vi "prepare_writing.vi"(8 "error in (no error)":errorcluster, 10 "fresh scan signals?":bool, 11 "DL090202ScanHead in":refnum<class "ScanHeadDL090202.lvclass">) -> (0 "error out":errorcluster, 3 "DL090202ScanHead out":refnum<class "ScanHeadDL090202.lvclass">)   [LabVIEW 2010, in "ScanHeadDL090202.lvclass"]
uses:
  ScanHeadDL090202.lvclass
  common/enumerations/functional_global_action_enum.ctl
  SignalWriter/GenericSignalWriter/GenericSignalWriter/GenericSignalWriter.lvclass
  Trajectory/TrajectoryDL091126GenericVoxel/TrajectoryDL091126GenericVoxel/TrajectoryDL091126GenericVoxel.lvclass
  ScanHeadDL090202.lvclass/ScanHeadDL090202.ctl
  Trajectory/GenericTrajectory/GenericTrajectory/GenericTrajectory.lvclass
  common/classes/GenericComponent/GenericComponent/class_data.vi
  common/classes/ErrorController/ErrorController/class_data.vi
  common/classes/ErrorController/ErrorController/ErrorController.lvclass
  common/classes/GenericComponent/GenericComponent/GenericComponent.lvclass
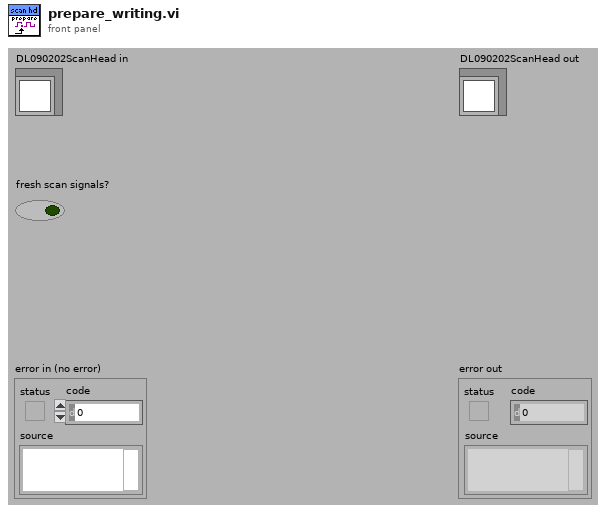
[diagram p1: front panel]
types:
  T1 = typedef "functional_global_action_enum.ctl" = enum16{"get", "set", "reset"}
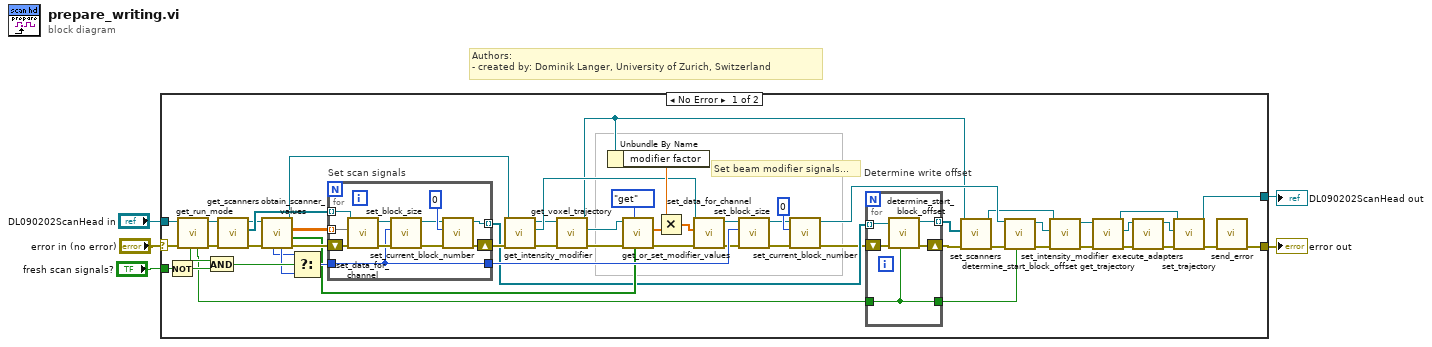
[diagram p0: block diagram]
diagram:
  # "Authors: \n- created by: Dominik Langer, University of Zurich, Switzerland"
  n1 = case shown="No Error" "error in (no error)" {
    selector: "error in (no error)" -> [w59 w80]
    tunnel: [w15 w80] -> w4
    tunnel: [w8 w79] -> w2
    tunnel: "DL090202ScanHead in" -> [w58 w79]
    tunnel: "fresh scan signals?" -> [w57 _]
    frame No Error {
      # "Set beam modifier signals..."
      n2 = Not(x=w57) -> (.not. x?=w55:bool)
      n3 = call "get_run_mode.vi"("error in (no error)"=w59, "GenericPlugin in"=w58) -> ("error out"=w31:errorcluster, "GenericPlugin out"=w30:refnum<class "ScanHeadDL090202.lvclass">, "is NOT free run?"=w51:bool, "is free run?"=w56:bool)  [unwired: 5 in, 1 out]
      n4 = And(x=w56, y=w55) -> (x .and. y?=w54:bool)
      n5 = call-dynamic "get_scanners.vi"("error in (no error)"=w31, "DL090202ScanHead.lvclass in"=w30) -> ("error out"=w34:errorcluster, "scanners"=w33:refnum<class "GenericSignalWriter.lvclass">[], "DL090202ScanHead.lvclass out"=w28:refnum<class "ScanHeadDL090202.lvclass">)  [unwired: 7 in]
      n6 = call-dynamic "obtain_scanner_values.vi"("error in (no error)"=w34, "ScanHeadDL090202 in"=w28) -> ("error out"=w50:errorcluster, "coerced?"=w46:bool[], "scan signals out"=w44:dbl[][], "ScanHeadDL090202 out"=w17:refnum<class "ScanHeadDL090202.lvclass">, "total number of pixels per cycle"=w49:i32, "block size"=w48:i32)  [unwired: 4 in]
      n7 = Select(t=w48, s=w54, f=w49) -> (s? t:f=w53:i32)
      n8 = for "Set scan signals" {
        shift-right: [w75] -> w24
        shift-left: w50 -> [w78]
        tunnel: w33 -> [w77] mode=indexing
        tunnel: w44 -> [w73] mode=indexing
        tunnel: [w74] -> w23 mode=indexing
        tunnel: w53 -> [w68]
        tunnel: [w68] -> w60
        n9 = call-dynamic "set_data_for_channel.vi"("error in (no error)"=w78, "data"=w73, "GenericWriteSignals in"=w77) -> ("error out"=w72:errorcluster, "GenericWriteSignals out"=w71:refnum<class "GenericSignalWriter.lvclass">)  [unwired: 7 out]
        n10 = call "set_block_size.vi"("error in (no error)"=w72, "block size (samples)"=w68, "GenericWriteSignals.lvclass in"=w71) -> ("error out"=w70:errorcluster, "GenericWriteSignals.lvclass out"=w69:refnum<class "GenericSignalWriter.lvclass">)  [unwired: 7 in]
        n11 = call-dynamic "set_current_block_number.vi"("error in (no error)"=w70, "current block number"=0, "GenericWriteSignals.lvclass in"=w69) -> ("error out"=w75:errorcluster, "GenericWriteSignals.lvclass out"=w74:refnum<class "GenericSignalWriter.lvclass">)  [unwired: 7 in]
      }
      n12 = call-dynamic "get_intensity_modifier.vi"("error in (no error)"=w24, "DL090202ScanHead.lvclass in"=w17) -> ("error out"=w29:errorcluster, "write signals"=w32:refnum<class "GenericSignalWriter.lvclass">, "DL090202ScanHead.lvclass out"=w27:refnum<class "ScanHeadDL090202.lvclass">)  [unwired: 7 in]
      n13 = call-dynamic "get_voxel_trajectory.vi"("error in (no error)"=w29, "ScanHeadDL090202 in"=w27) -> ("error out"=w47:errorcluster, "trajectory"=w45:refnum<class "TrajectoryDL091126GenericVoxel.lvclass">, "ScanHeadDL090202 out"=w16:refnum<class "ScanHeadDL090202.lvclass">)  [unwired: 7 in]
      n14 = Unbundle By Name(w16) -> ("modifier factor"=w62:dbl)
      n15 = call-dynamic "get_or_set_modifier_values.vi"("clamp output values?"=w46, "action"=functional_global_action_enum."get", "error in (no error)"=w47, "GenericTrajectory in"=w45) -> ("error out"=w38:errorcluster, "modifier values out"=w36:dbl[])  [unwired: 5 in, 1 out]
      n16 = Multiply(x=w62, y=w36) -> (x*y=w35:dbl[])
      n17 = call-dynamic "set_data_for_channel.vi"("error in (no error)"=w38, "data"=w35, "GenericWriteSignals in"=w32) -> ("error out"=w42:errorcluster, "GenericWriteSignals out"=w41:refnum<class "GenericSignalWriter.lvclass">)  [unwired: 7 out]
      n18 = call "set_block_size.vi"("error in (no error)"=w42, "block size (samples)"=w60, "GenericWriteSignals.lvclass in"=w41) -> ("error out"=w40:errorcluster, "GenericWriteSignals.lvclass out"=w39:refnum<class "GenericSignalWriter.lvclass">)  [unwired: 7 in]
      n19 = call-dynamic "set_current_block_number.vi"("error in (no error)"=w40, "current block number"=0, "GenericWriteSignals.lvclass in"=w39) -> ("error out"=w22:errorcluster, "GenericWriteSignals.lvclass out"=w61:refnum<class "GenericSignalWriter.lvclass">)  [unwired: 7 out]
      n20 = for "Determine write offset" {
        tunnel: w23 -> [w66] mode=indexing
        tunnel: [w65] -> w25 mode=indexing
        shift-right: [w64] -> w26
        shift-left: w22 -> [w67]
        tunnel: w51 -> [w63]
        tunnel: [w63] -> w52
        n21 = call-dynamic "determine_start_block_offset.vi"("force zero?"=w63, "error in (no error)"=w67, "GenericWriteSignals in"=w66) -> ("error out"=w64:errorcluster, "GenericWriteSignals out"=w65:refnum<class "GenericSignalWriter.lvclass">)  [unwired: 7 out]
      }
      n22 = call-dynamic "set_scanners.vi"("error in (no error)"=w26, "scanners"=w25, "DL090202ScanHead.lvclass in"=w16) -> ("error out"=w21:errorcluster, "DL090202ScanHead.lvclass out"=w18:refnum<class "ScanHeadDL090202.lvclass">)  [unwired: 7 in]
      n23 = call-dynamic "determine_start_block_offset.vi"("force zero?"=w52, "error in (no error)"=w21, "GenericWriteSignals in"=w61) -> ("error out"=w20:errorcluster, "GenericWriteSignals out"=w19:refnum<class "GenericSignalWriter.lvclass">)  [unwired: 7 out]
      n24 = call-dynamic "set_intensity_modifier.vi"("error in (no error)"=w20, "write signals"=w19, "DL090202ScanHead.lvclass in"=w18) -> ("error out"=w7:errorcluster, "DL090202ScanHead.lvclass out"=w9:refnum<class "ScanHeadDL090202.lvclass">)  [unwired: 7 in]
      n25 = call-dynamic "get_trajectory.vi"("error in (no error)"=w7, "GenericScanHead.lvclass in"=w9) -> ("error out"=w14:errorcluster, "trajectory"=w13:refnum<class "GenericTrajectory.lvclass">, "GenericScanHead.lvclass out"=w10:refnum<class "ScanHeadDL090202.lvclass">)  [unwired: 7 in]
      n26 = call-dynamic "execute_adapters.vi"("error in (no error)"=w14, "GenericTrajectory in"=w13) -> ("error out"=w12:errorcluster, "GenericTrajectory out"=w11:refnum<class "GenericTrajectory.lvclass">)  [unwired: 8 in]
      n27 = call-dynamic "set_trajectory.vi"("error in (no error)"=w12, "trajectory"=w11, "GenericScanHead.lvclass in"=w10) -> ("error out"=w6:errorcluster, "GenericScanHead.lvclass out"=w8:refnum<class "ScanHeadDL090202.lvclass">)  [unwired: 7 in]
      n28 = call "send_error.vi"("error in (no error)"=w6) -> ("error out"=w15:errorcluster)  [unwired: 10 in]
    }
    frame Error {
    }
  }
  "error out" <- w4
  "DL090202ScanHead out" <- w2
